vi "json Insert Float - array path.vi"(8 "error in (no error)":errorcluster, 9 "anything":sgl, 10 "path":string[](array[string]), 11 "JSON Document in":refnum<class "JSON Document.lvclass">) -> (0 "error out":errorcluster, 2 "replaced?":bool, 3 "JSON Document out":refnum<class "JSON Document.lvclass">)   [LabVIEW 2015, in "JSON Document.lvclass"]
uses:
  JSON Document.lvclass
  json Insert Float - string path.vi
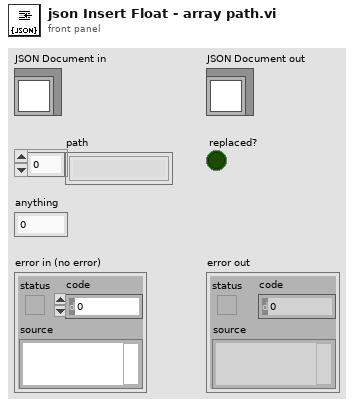
[diagram p1: front panel]
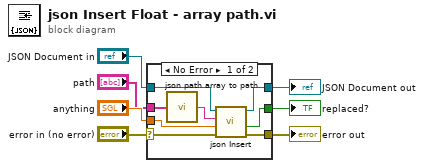
[diagram p0: block diagram]
diagram:
  n1 = case shown="No Error" "error in (no error)" {
    selector: "error in (no error)" -> [w9 w17]
    tunnel: [w13 w17] -> w6
    tunnel: [w12 w16] -> w4
    tunnel: "JSON Document in" -> [w11 w16]
    tunnel: "anything" -> [w10 _]
    tunnel: "path" -> [w14 _]
    tunnel: [w8 _] -> w1
    frame No Error {
      n2 = call "json path array to path.vi"("path"=w14) -> ("String"=w15:string)
      n3 = call-poly "json Insert.vi"("error in (no error)"=w9, "anything"=w10, "path"=w15, "JSON Document in"=w11) -> ("error out"=w13:errorcluster, "replaced?"=w8:bool, "JSON Document out"=w12:refnum<class "JSON Document.lvclass">)  [unwired: 5 in]
    }
    frame Error {
    }
  }
  "error out" <- w6
  "JSON Document out" <- w4
  "replaced?" <- w1
